vi "Reset All Colours.vi"(8 "error in (no error)":errorcluster, 11 "Hex Viewer in":refnum<class "Hex Viewer.lvclass">) -> (0 "error out":errorcluster)   [LabVIEW 2021, in "Hex Viewer.lvclass"]
uses:
  Hex Viewer.lvclass
  <vilib>/Utility/miscctls.llb/LVRowAndColumnTypeDef.ctl
  Hex Viewer.lvclass/Hex Viewer.ctl
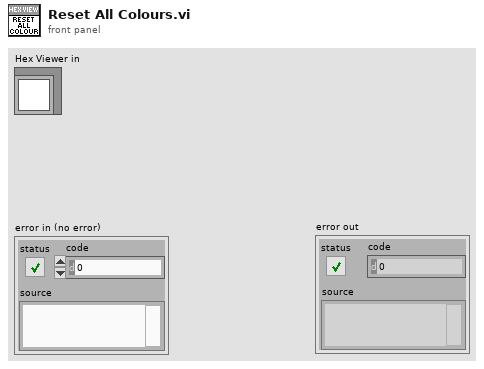
[diagram p1: front panel]
types:
  T1 = typedef "LVRowAndColumnTypeDef.ctl" = cluster{"Row":i32, "Column":i32}
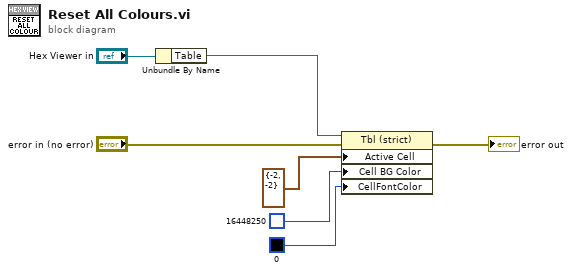
[diagram p0: block diagram]
diagram:
  n1 = Unbundle By Name("Hex Viewer in") -> ("Table"=w6:refnum<vi>)
  n2 = property class="Tbl (strict)"(reference=w6, error in="error in (no error)", "Active Cell"=T1 {"Row"=-2, "Column"=-2} ("Active Cell:Active Cell"), "Cell BG Color"=u32 16448250 ("Active Cell:Cell Background Color"), "CellFontColor"=u32 0 ("Active Cell:Cell Font:Color")) -> (error out=→"error out":errorcluster)  [unwired: 1 out]
